vi "Pre-Build Custom Action_cli_lv_systemexec_poc.vi"(10 "Variant":variant) -> (0 "error out":errorcluster)   [LabVIEW 2021]
panel:
  out "Numeric":i32
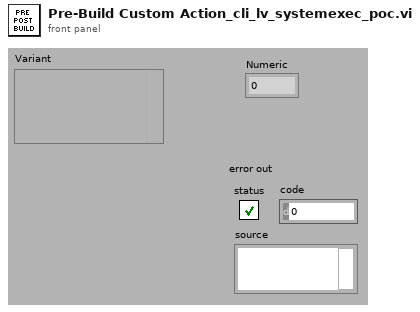
[diagram p1: front panel]
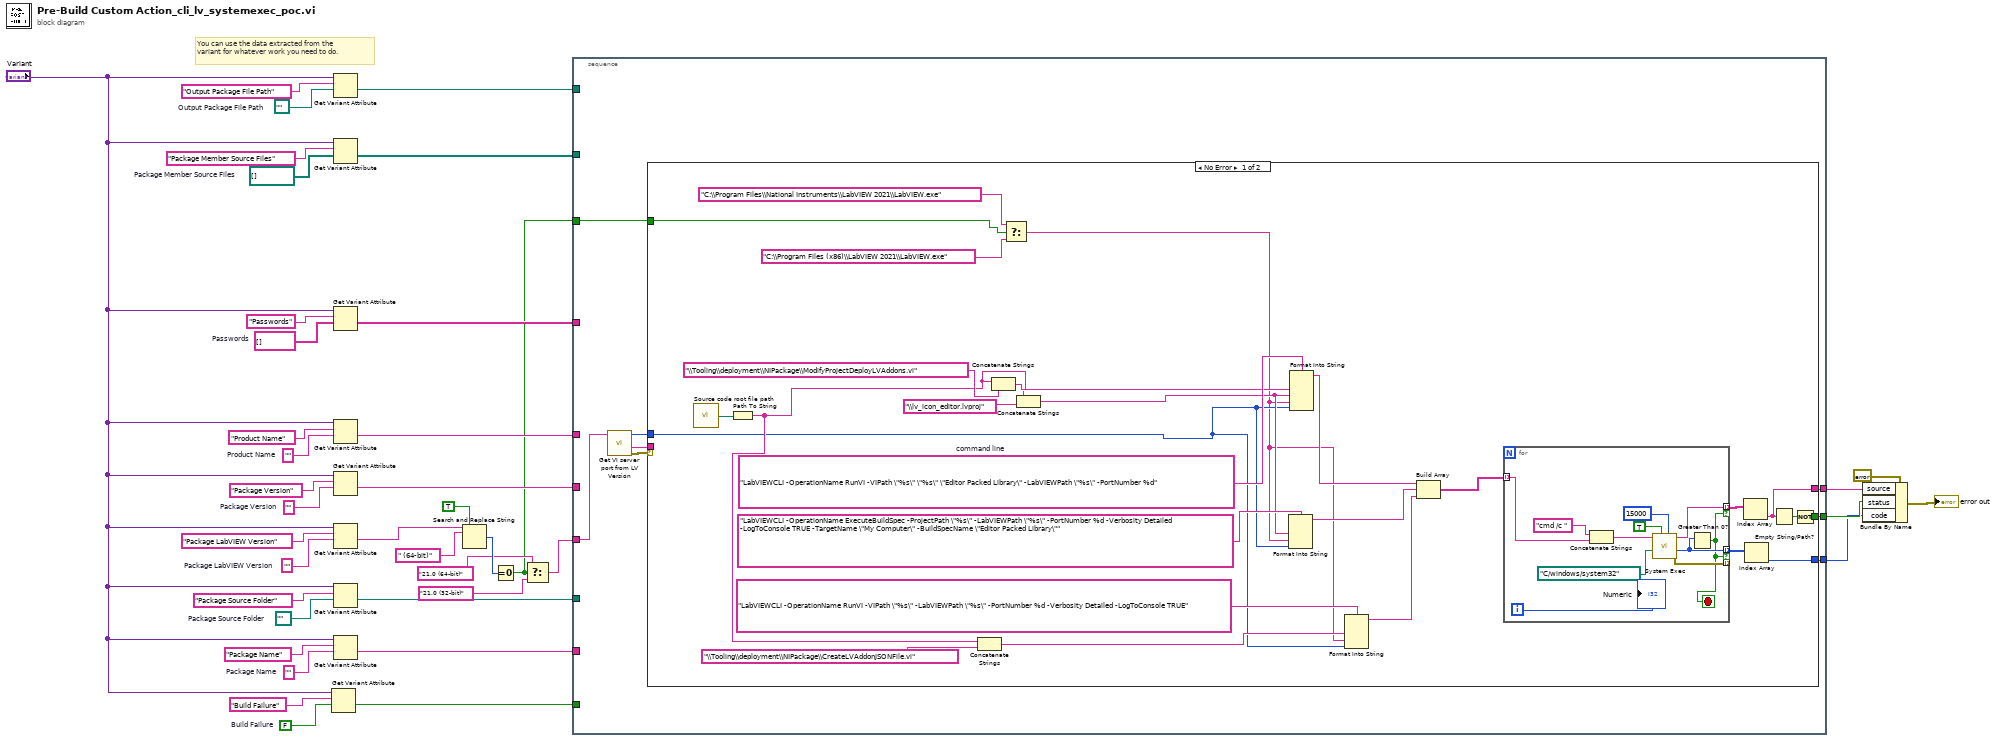
[diagram p0: block diagram]
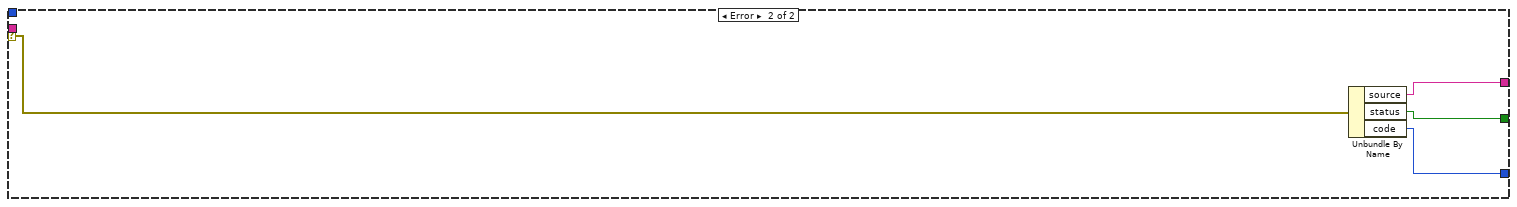
[diagram p2: hidden frame]
diagram:
  w16 = FALSE  # Build Failure
  w25 = path ""  # Package Source Folder
  w26 = ""  # Package Name
  w29 = ""  # Package LabVIEW Version
  w31 = ""  # Package Version
  w33 = ""  # Product Name
  w35 = string[] []  # Passwords
  w37 = path[] []  # Package Member Source Files
  w39 = path ""  # Output Package File Path
  # "You can use the data extracted from the variant for whatever work you need to do."
  n1 = Get Variant Attribute(Variant="Variant", name="Build Failure", default value (empty Variant)=w16) -> (value=w14:bool)  [unwired: 1 in, 3 out]
  n2 = Get Variant Attribute(Variant="Variant", name="Output Package File Path", default value (empty Variant)=w39) -> (value=w24:path)  [unwired: 1 in, 3 out]
  n3 = Get Variant Attribute(Variant="Variant", name="Package Member Source Files", default value (empty Variant)=w37) -> (value=w23:path[])  [unwired: 1 in, 3 out]
  n4 = Get Variant Attribute(Variant="Variant", name="Passwords", default value (empty Variant)=w35) -> (value=w22:string[])  [unwired: 1 in, 3 out]
  n5 = Get Variant Attribute(Variant="Variant", name="Product Name", default value (empty Variant)=w33) -> (value=w21:string)  [unwired: 1 in, 3 out]
  n6 = Get Variant Attribute(Variant="Variant", name="Package Version", default value (empty Variant)=w31) -> (value=w20:string)  [unwired: 1 in, 3 out]
  n7 = Get Variant Attribute(Variant="Variant", name="Package LabVIEW Version", default value (empty Variant)=w29) -> (value=w6:string)  [unwired: 1 in, 3 out]
  n8 = Get Variant Attribute(Variant="Variant", name="Package Source Folder", default value (empty Variant)=w25) -> (value=w19:path)  [unwired: 1 in, 3 out]
  n9 = Get Variant Attribute(Variant="Variant", name="Package Name", default value (empty Variant)=w26) -> (value=w18:string)  [unwired: 1 in, 3 out]
  n10 = Search and Replace String(replace all?=TRUE ("replace all? (F)"), input string=w6, search string=" (64-bit)") -> (number of replacements=w5:i32)  [unwired: 5 in, 3 out]
  n11 = Equal To 0?(x=w5) -> (x = 0?=w1:bool)
  n12 = Select(t="21.0 (64-bit)", s=w1, f="21.0 (32-bit)") -> (s? t:f=w2:string)
  n13 = stacked-sequence {
    tunnel: w24 -> [_]
    tunnel: w23 -> [_]
    tunnel: w22 -> [_]
    tunnel: w21 -> [_]
    tunnel: w20 -> [_]
    tunnel: w2 -> [w42]
    tunnel: w19 -> [_]
    tunnel: w18 -> [_]
    tunnel: w14 -> [_]
    tunnel: [w48] -> w12
    tunnel: [w47] -> w11
    tunnel: [w46] -> w10
    tunnel: w1 -> [w41]
    frame #0 {
      n14 = call "Get VI server port from LV Version.vi"("input string"=w42) -> ("error out"=w43:errorcluster, "LabVIEW path"=w45:string, "VI Server port"=w44:u32)  [unwired: 7 in, 1 out]
      n15 = case shown="No Error" w43 {
        selector: w43 -> [_ w89]
        tunnel: [w71 w87] -> w48
        tunnel: [w69 w86] -> w47
        tunnel: [w68 w88] -> w46
        tunnel: w45 -> [_ _]
        tunnel: w44 -> [w54 _]
        tunnel: w41 -> [w49 _]
        frame No Error {
          w67 = "LabVIEWCLI -OperationName RunVI -VIPath \"%s\" \"%s\" \"Editor Packed Library\" -LabVIEWPath \"%s\" -PortNumber %d"  # command line
          n16 = call "Source code root file path.vi"() -> ("Source code root path"=w53:path)  [unwired: 1 in]
          n17 = Path To String(path=w53) -> (string=w57:string)
          n18 = Concatenate Strings(w57, "\\Tooling\\deployment\\NIPackage\\CreateLVAddonJSONFile.vi" ("string")) -> (w55:string)
          n19 = Concatenate Strings(w57, "\\Tooling\\deployment\\NIPackage\\ModifyProjectDeployLVAddons.vi" ("input 1")) -> (w62:string)
          n20 = Select(t="C:\\Program Files\\National Instruments\\LabVIEW 2021\\LabVIEW.exe" ("input string"), s=w49, f="C:\\Program Files (x86)\\LabVIEW 2021\\LabVIEW.exe" ("input string")) -> (s? t:f=w50:string)
          n21 = Concatenate Strings(w57, "\\lv_icon_editor.lvproj" ("input 2")) -> (w60:string)
          n22 = Format Into String(format string="LabVIEWCLI -OperationName ExecuteBuildSpec -ProjectPath \"%s\" -LabVIEWPath \"%s\" -PortNumber %d -Verbosity Detailed -LogToConsole TRUE -TargetName \"My Computer\" -BuildSpecName \"Editor Packed Library\"" ("command line"), w60, w50, w54) -> (resulting string=w64:string)  [unwired: 2 in, 1 out]
          n23 = Format Into String(format string=w67, w62, w60, w50, w54) -> (resulting string=w66:string)  [unwired: 2 in, 1 out]
          n24 = Format Into String(format string="LabVIEWCLI -OperationName RunVI -VIPath \"%s\" -LabVIEWPath \"%s\" -PortNumber %d -Verbosity Detailed -LogToConsole TRUE" ("command line"), w55, w50, w54) -> (resulting string=w58:string)  [unwired: 2 in, 1 out]
          n25 = Build Array(w66, w64, w58) -> (w74:string[])
          n26 = for {
            tunnel: w74 -> [w82] mode=indexing
            tunnel: [w81] -> _ mode=indexing
            tunnel: [w78] -> w70 mode=indexing if=w75
            tunnel: [w77] -> w73 mode=indexing if=w75
            i -> [w80]
            stop <- w75 stop-if-true
            n27 = Concatenate Strings("cmd /c " ("command line"), w82) -> (w84:string)
            n28 = call <vilib>:"System Exec.vi"("expected output size  (4096)"=u32 15000, "wait until completion? (T)"=TRUE, "working directory"=path "C:/windows/system32", "command line"=w84) -> ("error out"=w81:errorcluster, "return code"=w78:i32, "standard output"=w77:string)  [unwired: 4 in, 1 out]
            n29 = Greater Than 0?(x=w78) -> (x > 0?=w75:bool)
            "Numeric" <- w80
          }
          n30 = Index Array(array=w73) -> (element=w68:string)  [unwired: 1 in]
          n31 = Index Array(array=w70) -> (element=w69:i32)  [unwired: 1 in]
          n32 = Empty String/Path?(string/path=w68) -> (empty?=w72:bool)
          n33 = Not(x=w72) -> (.not. x?=w71:bool)
        }
        frame Error {
          n34 = Unbundle By Name(w89) -> ("source"=w88:string, "status"=w87:bool, "code"=w86:i32)
        }
      }
    }
  }
  n35 = Bundle By Name(cluster=errorcluster {"status"=FALSE, "code"=0, "source"=""} ("error out"), "source"=w10, "status"=w12, "code"=w11) -> (→"error out":errorcluster)
